vi "Overlay LineOut from ROI XDisplay.vi"(0 "Image In":T3, 1 "ROI":T1, 3 "Calbration":dbl=1.0, 4 "Group":string, 5 "error in":errorcluster) -> (6 "Image Out":T3, 7 "FWHM":dbl[](array[numeric]), 8 "error out":errorcluster)   [LabVIEW 2020, in "POLARIS IMAQ Display.xctl"]
doc: "Filters ROI countours of line type and shows their lineotus like a trend with arbitary units. If slope of the line is les 45° trend appears at bottom border otherwise at the left border. \n\nthanks for idee and first implementation to Sebastian Keppler, FSU-IOQ\n\nauthor: Alexander Kessler, Helmholtz-Institut-Jena \nmaintainer: Alexander Kessler: alexander.kessler@uni-jena.de\n\n\n\nLicense Agreement for this software:\n\nCopyright (C)\nHelmholtz-Institut-Jena\nFröbelstieg 3\n07743 Jena\nGermany\n\nThis program is free software; you can redistribute it and/or modify it under the terms of the GNU General Public License as published by the Free Software Foundation; either version 2 of the license, or (at your option) any later version.\n\nThis program is distributed in the hope that it will be useful, but WITHOUT ANY WARRANTY; without even the implied warranty of MERCHANTABILITY or FITNESS FOR A PARTICULAR PURPOSE. See the GNU General License for more details (http://www.gnu.org)."
uses:
  POLARIS IMAQ Display.xctl
  <vilib>/vision/Image Controls.llb/IMAQ Image.ctl
panel:
  out "Waveform Graph":T2(graph)
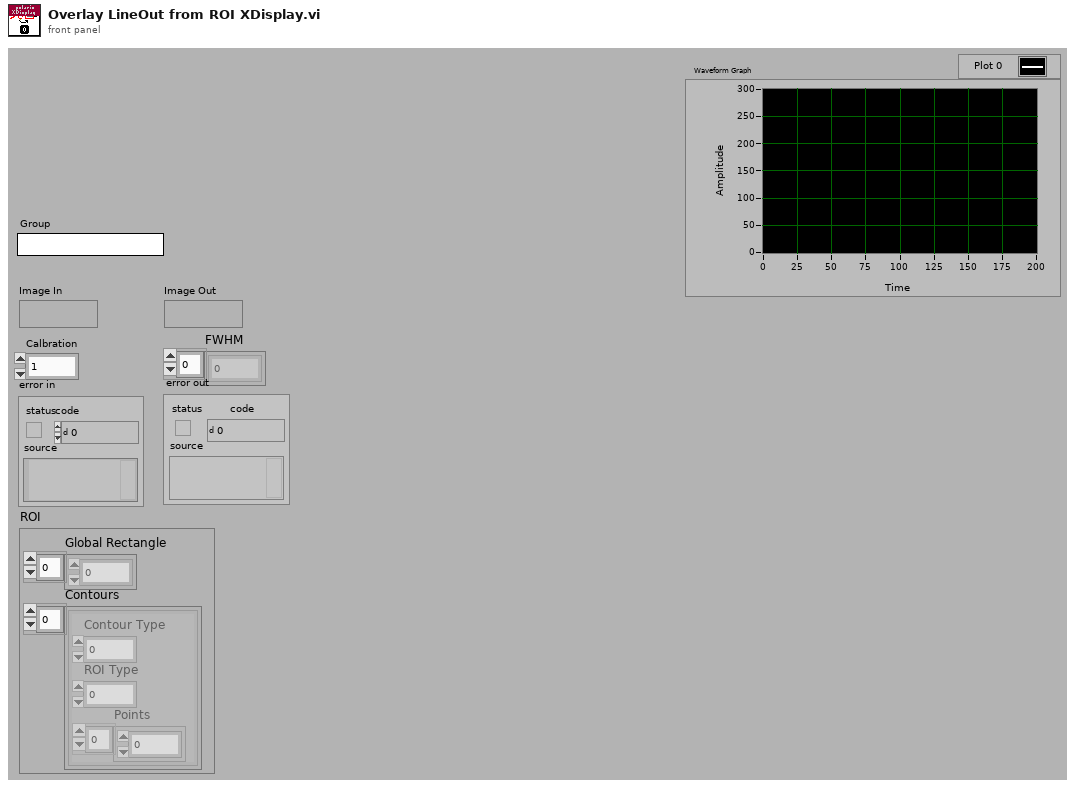
[diagram p1: front panel]
types:
  T1 = cluster{"Global Rectangle":i32[], "Contours":cluster{"Contour Type":u32, "ROI Type":u32, "Points":i32[]}[]}
  T2 = cluster{"x0":sgl, "dx":sgl, "Pixels Line":sgl[]}[]
  T3 = typedef "IMAQ Image.ctl" = refnum<image>
  T4 = cluster{"Contour Type":u32, "ROI Type":u32, "Points":i32[]}[]
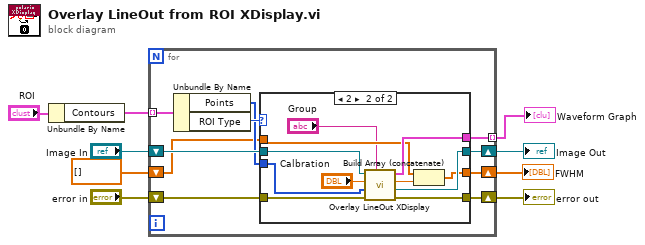
[diagram p0: block diagram]
diagram:
  n1 = Unbundle By Name("ROI") -> ("Contours"=w9:T4)
  n2 = for {
    tunnel: w9 -> [w19] mode=indexing
    tunnel: [w15] -> w8 mode=indexing
    shift-right: [w14] -> w5
    shift-left: "Image In" -> [w17]
    shift-right: [w12] -> w4
    shift-left: dbl[] [] -> [w13]
    shift-right: [w10] -> w1
    shift-left: "error in" -> [w11]
    n3 = Unbundle By Name(w19) -> ("Points"=w16:i32[], "ROI Type"=w18:u32)
    n4 = case shown="2" w18 {
      tunnel: w17 -> [w22 w33]
      tunnel: w16 -> [_ w31]
      tunnel: [_ w30] -> w15
      tunnel: [w22 w32] -> w14
      tunnel: w13 -> [w21 w29]
      tunnel: [w21 w28] -> w12
      tunnel: w11 -> [w20 w25]
      tunnel: [w20 w24] -> w10
      frame 0, Default {
      }
      frame 2 {
        n5 = call "Overlay LineOut XDisplay.vi"("Group"="Group", "error in"=w25, "LineCoord"=w31, "Calibration"="Calbration", "Image In"=w33) -> ("error out"=w24:errorcluster, "Image Out"=w32:T3, "FWHM"=w26:dbl, "Line Graph"=w30:cluster{"x0":sgl, "dx":sgl, "Pixels Line":sgl[]})  [unwired: 3 in]
        n6 = Build Array (concatenate)(w29, w26) -> (w28:dbl[])
      }
    }
  }
  "Image Out" <- w5
  "Waveform Graph" <- w8
  "FWHM" <- w4
  "error out" <- w1
